vi "Number.vi"(8 "Error In":errorcluster, 10 "Number":dbl, 11 "TestLNA in":refnum<class "TestLNA.lvclass">) -> (0 "Error Out":errorcluster, 3 "TestLNA out":refnum<class "TestLNA.lvclass">)   [LabVIEW 2016, in "TestLNA.lvlib" / "TestLNA.lvclass"]
doc: "Set number to attribute and display in dialog."
uses:
  TestLNA.lvclass
  C:/User/Brand/LVP/CSPP-Dev/Packages/CSPP_Core/Actors/CS++BaseActor/CS++BaseActor.lvclass
  TestLNA.lvclass/TestLNA.ctl
  CSPP_Core/Actors/CS++BaseActor/CS++BaseActor.lvclass/CS++BaseActor.ctl
  CSPP_Core/Actors/CS++BaseActor/Read Object Name.vi
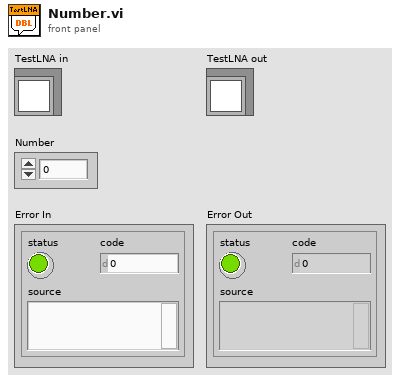
[diagram p1: front panel]
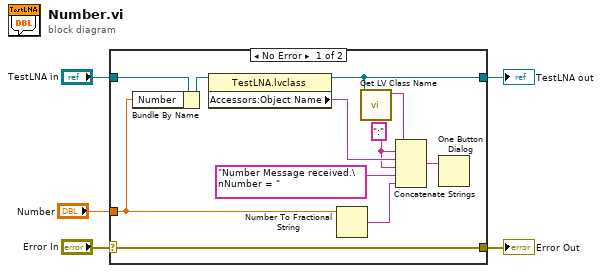
[diagram p0: block diagram]
diagram:
  n1 = case shown="No Error" "Error In" {
    selector: "Error In" -> [w16 w18]
    tunnel: [w16 w18] -> w4
    tunnel: [w10 w17] -> w2
    tunnel: "TestLNA in" -> [w8 w17]
    tunnel: "Number" -> [w6 _]
    frame No Error {
      w11 = ":" ("string")
      n2 = Bundle By Name(cluster=w8, "Number"=w6) -> (w7:refnum<class "TestLNA.lvclass">)
      n3 = property class="TestLNA.lvclass"(reference=w7) -> (reference out=w10:refnum<class "TestLNA.lvclass">, "Accessors:Object Name"=w12:string)  [unwired: 1 in, 1 out]
      n4 = Number To Fractional String(number=w6) -> (F-format string=w9:string)  [unwired: 3 in]
      n5 = call <vilib>:"Get LV Class Name.vi"("object"=w10) -> ("class name"=w13:string)  [unwired: 9 in, 1 out]
      n6 = Concatenate Strings(w13, w11, w12, w11, "Number Message received.\nNumber = " ("message"), w9) -> (w14:string)
      n7 = One Button Dialog(message=w14) -> ()  [unwired: 1 in, 1 out]
    }
    frame Error {
    }
  }
  "Error Out" <- w4
  "TestLNA out" <- w2
